vi "NF87XX.get Driver.vi"(0 "i ref in":refnum<vi>, 2 "System":string="N/A", 5 "error in (no error)":errorcluster) -> (14 "i ref out":refnum<vi>, 16 "Driver Type":T1, 17 "Driver":string, 18 "Driver Index":i32, 19 "error out":errorcluster)   [LabVIEW 2014, in "NF87XX.lvlib"]
doc: "Within this VI the Driver is figured out. Thereby \"System\" is either the name or the driver: if \"System\" is looking like \"Axx\" where \"xx\" stands for one or two characters, \"System is directly coming out as Driver. Otherwise the ingoing \"System\" is compared with the names sotred in own attributes and thereby the driver is given out. If nothing of this is true, \"N/A\" is given out. \nIt also gives out the Driver Type of the driver.\n\nauthor: Stefan Götte\ndata: 09-JAN-2007"
uses:
  NF87XX.lvlib
  NF87XX.driver Type.ctl
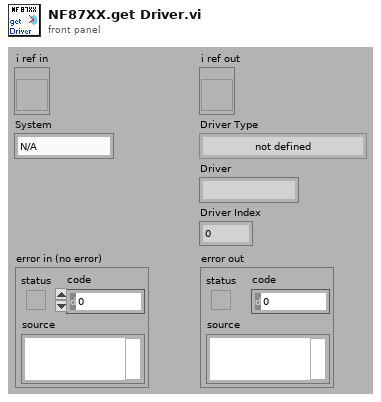
[diagram p1: front panel]
types:
  T1 = typedef "NF87XX.lvlib/NF87XX.driver Type.ctl" = enum16{"not defined", "3-ch open loop drv", "1-ch closed loop drv"}
  T2 = typedef "NF87XX.lvlib/NF87XX.i attribute.ctl" = cluster{"Con Settings":T3, "Drivers":T4[], "Status":cluster{"Service ID":i32, "Status":T6}, "Joystick available":bool, "VISA Resource":string}
  T3 = typedef "NewFocusPico - Driver np.lvlib/VISA & TCPIP Control.ctl" = cluster{"VISA or TCP/IP":bool, "Init Connection":bool, "Close Connection":bool, "Resource Name":refnum<visa-resource-name>, "hostname":string, "connection ID":refnum<k5>}
  T4 = typedef "NF87XX.lvlib/NF87XX.driver Settings.ctl" = cluster{"Name":string, "Driver Type":T1, "Pico Parameter type":T5, "Acceleration [Steps/s²]":cluster{"Motor 0":dbl, "Motor 1":dbl, "Motor 2":dbl}, "Start Velocity [Steps/s]":cluster{"Motor 0":dbl, "Motor 1":dbl, "Motor 2":dbl}, "Velocity [Steps/s]":cluster{"Motor 0":dbl, "Motor 1":dbl, "Motor 2":dbl}, "axis channel":i32, "Position":i32, "Position Service ID":i32}
  T5 = typedef "NewFocusPico - Driver np.lvlib/Pico Parameters.ctl" = cluster{"Pico Type":enum16{"Open-Loop Pico", "Close-Loop Pico", "Pico Ultra"}, "Acceleration (steps/sec^2)":string, "Velocity ( Hz)":string, "Driver":string, "Motor":string, "Channel":string, "Process Step":string}
  T6 = typedef "PH_StatusHandler.lvlib/PH_StatusHandler.Status.ctl" = i16
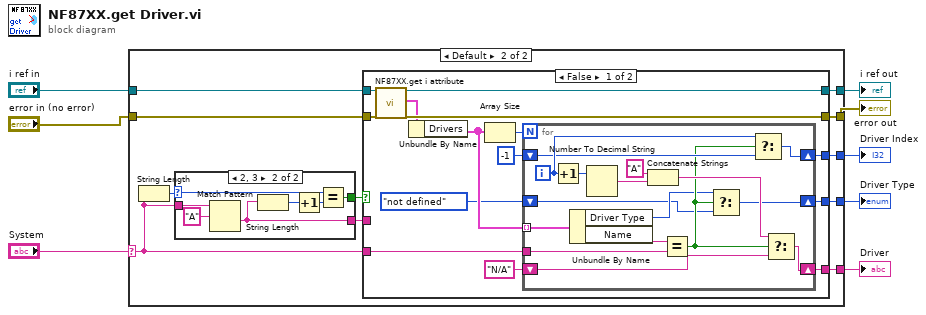
[diagram p0: block diagram]
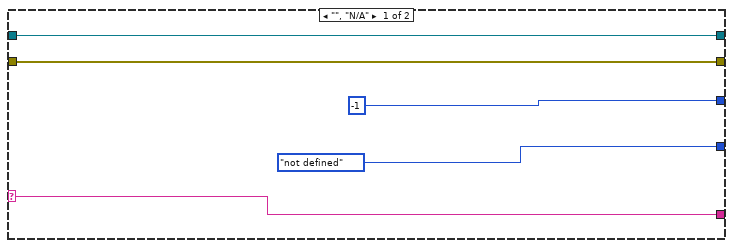
[diagram p2: hidden frame]
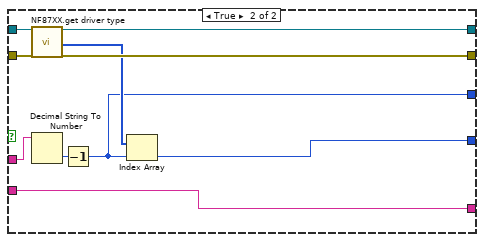
[diagram p3: hidden frame]
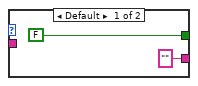
[diagram p4: hidden frame]
diagram:
  n1 = case shown="Default" "System" {
    selector: "System" -> [w13 w18]
    tunnel: [w13 w24] -> w8
    tunnel: [w12 w23] -> w7
    tunnel: "error in (no error)" -> [w12 w22]
    tunnel: [w11 w21] -> w5
    tunnel: "i ref in" -> [w11 w20]
    tunnel: [NF87XX.driver_Type."not defined" ("Driver Type") w16] -> w2
    tunnel: [-1 w14] -> w1
    frame "", "N/A" {
    }
    frame Default {
      n2 = String Length(string=w18) -> (length=w19:i32)
      n3 = case shown="2, 3" w19 {
        selector: w19 -> [_ w71]
        tunnel: w18 -> [_ w73]
        tunnel: [FALSE w68] -> w17
        tunnel: ["" w67] -> w15
        frame Default {
        }
        frame 2, 3 {
          n4 = Match Pattern(string=w73, regular expression="A") -> (after substring=w67:string)  [unwired: 1 in, 3 out]
          n5 = String Length(string=w67) -> (length=w70:i32)
          n6 = Increment(x=w70) -> (x+1=w69:i32)
          n7 = Equal?(x=w71, y=w69) -> (x = y?=w68:bool)
        }
      }
      n8 = case shown="False" w17 {
        tunnel: [w38 w64] -> w24
        tunnel: [w37 w60] -> w23
        tunnel: w22 -> [w36 w61]
        tunnel: [w35 w62] -> w21
        tunnel: w20 -> [w34 w63]
        tunnel: w18 -> [w29 w64]
        tunnel: [w28 w56] -> w16
        tunnel: w15 -> [_ w59]
        tunnel: [w27 w55] -> w14
        frame False {
          n9 = call "NF87XX.get i attribute.vi"("i ref in"=w34, "error in (no error)"=w36) -> ("i ref out"=w35:refnum<vi>, "i attribute"=w33:T2, "error out"=w37:errorcluster)  [unwired: 15 in]
          n10 = Unbundle By Name(w33) -> ("Drivers"=w30:T4[])
          n11 = Array Size(array=w30) -> (size(s)=w32:i32)
          n12 = for {
            N: w32 -> [_]
            tunnel: w30 -> [w53] mode=indexing
            shift-right: [w50] -> w38
            shift-left: "N/A" -> [w49]
            tunnel: w29 -> [w52]
            shift-right: [w42] -> w28
            shift-left: NF87XX.driver_Type."not defined" ("Driver Type") -> [w39]
            shift-right: [w44] -> w27
            shift-left: -1 -> [w43]
            i -> [w45]
            n13 = Increment(x=w45) -> (x+1=w48:i32)
            n14 = Unbundle By Name(w53) -> ("Driver Type"=w40:T1, "Name"=w54:string)
            n15 = Number To Decimal String(number=w48) -> (decimal integer string=w46:string)  [unwired: 1 in]
            n16 = Concatenate Strings("A" ("string"), w46) -> (w51:string)
            n17 = Equal?(x=w54, y=w52) -> (x = y?=w41:bool)
            n18 = Select(t=w40, s=w41, f=w39) -> (s? t:f=w42:T1)
            n19 = Select(t=w45, s=w41, f=w43) -> (s? t:f=w44:i32)
            n20 = Select(t=w51, s=w41, f=w49) -> (s? t:f=w50:string)
          }
        }
        frame True {
          n21 = call "NF87XX.get driver type.vi"("i ref in"=w63, "error in (no error)"=w61) -> ("i ref out"=w62:refnum<vi>, "Driver Types"=w57:T1[], "error out"=w60:errorcluster)  [unwired: 15 in]
          n22 = Decimal String To Number(string=w59) -> (number=w58:i32)  [unwired: 2 in, 1 out]
          n23 = Decrement(x=w58) -> (x-1=w55:i32)
          n24 = Index Array(array=w57, index=w55) -> (element=w56:T1)
        }
      }
    }
  }
  "Driver" <- w8
  "error out" <- w7
  "i ref out" <- w5
  "Driver Type" <- w2
  "Driver Index" <- w1
